vi "Check Error and Get Call Result.vi"(8 "error in (no error)":errorcluster, 10 "Response body":string, 11 "Response header":string) -> (0 "error out":errorcluster, 1 "Redirect endpoint":string, 2 "500 Or Throttled?":bool=TRUE, 3 "Call Result":string)   [LabVIEW 2015, in "NI_AWS Core.lvlib"]
doc: "Check the respnse header and body if necessary to obtain the call's result (Success or Error codes)."
uses:
  NI_AWS Core.lvlib
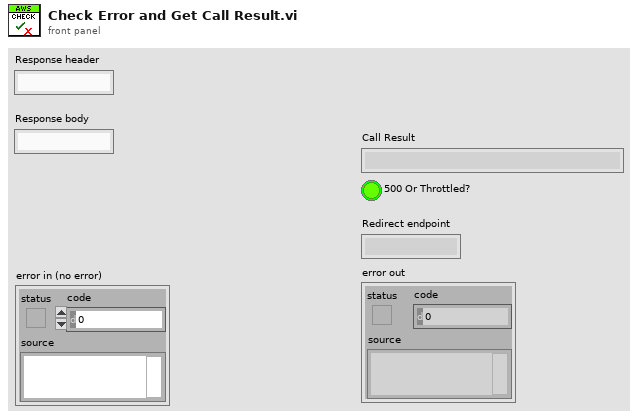
[diagram p1: front panel]
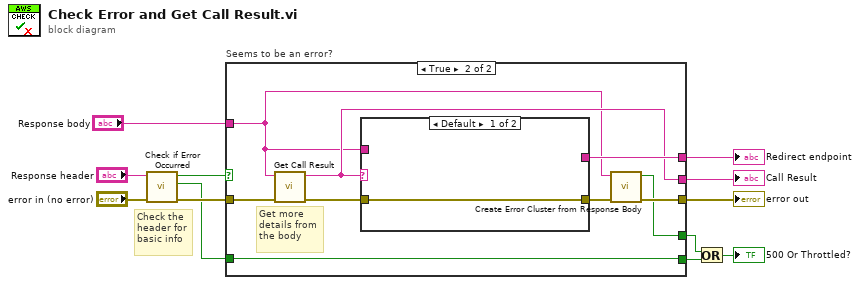
[diagram p0: block diagram]
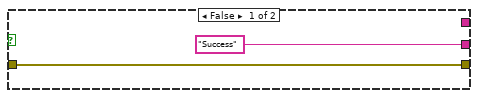
[diagram p2: hidden frame]
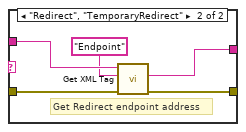
[diagram p3: hidden frame]
diagram:
  # "Check the\nheader for\nbasic info"
  n1 = call "Check if Error Occurred.vi"("error in (no error)"="error in (no error)", "Response header"="Response header") -> ("error out"=w9:errorcluster, "500 Error?"=w4:bool, "Error Occured?"=w10:bool)  [unwired: 7 in]
  n2 = case "Seems to be an error?" shown="True" w10 {
    tunnel: w9 -> [w14 w23]
    tunnel: "Response body" -> [_ w17]
    tunnel: [w14 w18] -> w6
    tunnel: ["Success" ("Call Result") w21] -> w7
    tunnel: [_ w22] -> w5
    tunnel: [_ w16] -> w1
    tunnel: [_ w15] -> w3
    tunnel: w4 -> [_ w15]
    frame False {
    }
    frame True {
      # "Get more\ndetails from\nthe body"
      n3 = call "Get Call Result.vi"("error in (no error)"=w23, "Response body"=w17) -> ("error out"=w20:errorcluster, "Call Result"=w21:string)  [unwired: 8 in]
      n4 = case shown="Default" w21 {
        tunnel: w17 -> [_ w29]
        tunnel: [_ w27] -> w22
        tunnel: [w24 w26] -> w19
        tunnel: w20 -> [w24 w25]
        frame Default {
        }
        frame "Redirect", "TemporaryRedirect" {
          # "Get Redirect endpoint address"
          n5 = call "Get XML Tag.vi"("error in (no error)"=w25, "Tag name"="Endpoint", "XML String in"=w29) -> ("error out"=w26:errorcluster, "Tag value"=w27:string)  [unwired: 4 in, 3 out]
        }
      }
      n6 = call "Create Error Cluster from Response Body.vi"("error in (no error)"=w19, "Response body"=w17) -> ("error out"=w18:errorcluster, "Is Throttled?"=w16:bool)  [unwired: 8 in]
    }
  }
  "Call Result" <- w7
  "error out" <- w6
  "Redirect endpoint" <- w5
  n7 = Or(x=w1, y=w3) -> (x .or. y?=→"500 Or Throttled?":bool)
